vi "rotate string.vi"() -> ()   [LabVIEW 2020]
panel:
  in  "stop":bool
  out "String":string
  in  "Enter a String":string
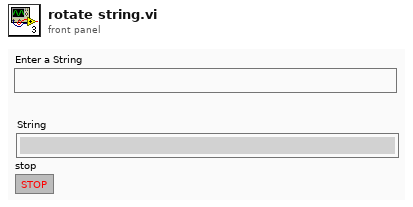
[diagram p1: front panel]
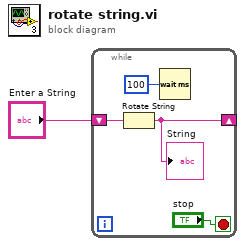
[diagram p0: block diagram]
diagram:
  n1 = while {
    shift-right: [w4] -> _
    shift-left: "Enter a String" -> [w5]
    stop <- "stop" stop-if-true
    n2 = Rotate String(1:w5) -> (0:w4:string)
    "String" <- w4
    n3 = Wait (ms)(milliseconds to wait=u32 100) -> ()  [unwired: 1 out]
  }
